vi "RichToFlatni_measurementlink_pinmap_v1_PinDefinition.vi"(5 "OutputClusterType":T1, 11 "InputCluster":T2) -> (3 "OutputCluster":T1)   [LabVIEW 2020, in "MeasurementLink Pin Map Client.lvlib"]
uses:
  MeasurementLink Pin Map Client.lvlib
  ni_measurementlink_pinmap_v1_PinDefinition.ctl
  ni_measurementlink_pinmap_v1_PinDefinition_Flat.ctl
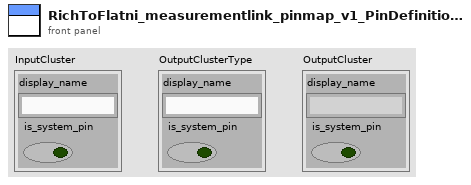
[diagram p1: front panel]
types:
  T1 = typedef "MeasurementLink Pin Map Client.lvlib/ni_measurementlink_pinmap_v1_PinDefinition_Flat.ctl" = cluster{"display_name":string, "is_system_pin":bool}
  T2 = typedef "MeasurementLink Pin Map Client.lvlib/ni_measurementlink_pinmap_v1_PinDefinition.ctl" = cluster{"display_name":string, "is_system_pin":bool}
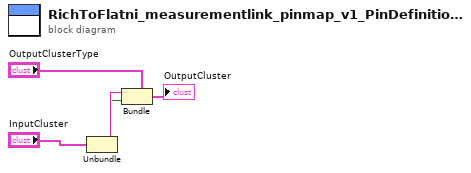
[diagram p0: block diagram]
diagram:
  n1 = Unbundle "Unbundle"("InputCluster") -> ("display_name"=w2:string, "is_system_pin"=w1:bool)
  n2 = Bundle "Bundle"(cluster="OutputClusterType", "display_name"=w2, "is_system_pin"=w1) -> (→"OutputCluster":T1)
